vi "ContinousTest.vi"() -> ()   [LabVIEW 2020]
uses:
  <vilib>/Analysis/NI_AALBase.lvlib
  source/library/openg_md5.lvlib
  source/library/MD5 Message Digest/MD5 Message Digest (Binary String).vi
panel:
  out "Iteration":i32
  out "All OK?":bool
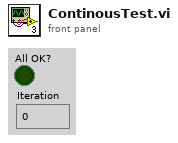
[diagram p1: front panel]
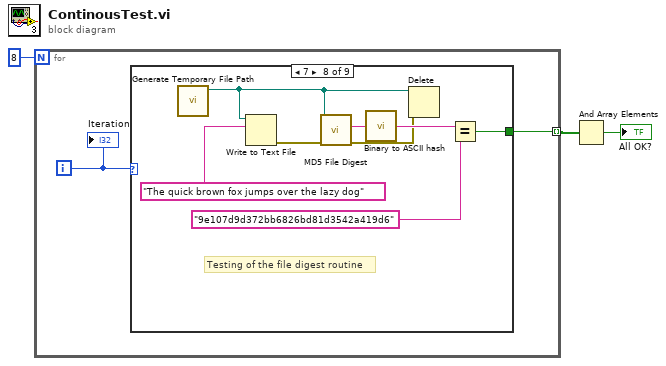
[diagram p0: block diagram]
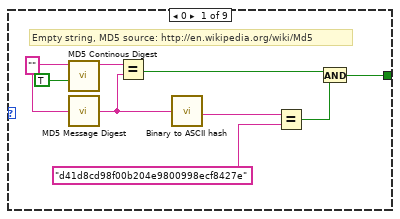
[diagram p2: hidden frame]
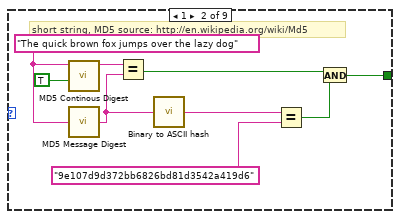
[diagram p3: hidden frame]
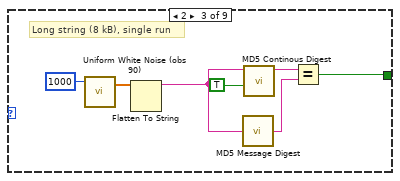
[diagram p4: hidden frame]
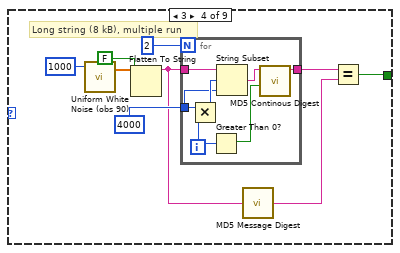
[diagram p5: hidden frame]
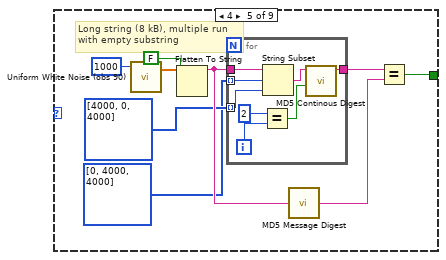
[diagram p6: hidden frame]
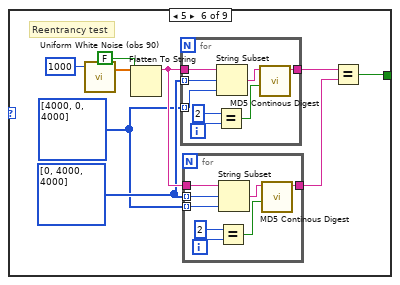
[diagram p7: hidden frame]
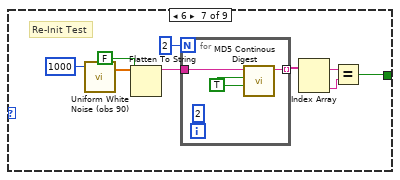
[diagram p8: hidden frame]
diagram:
  n1 = for {
    N: 8 -> [_]
    tunnel: [w4] -> w2 mode=indexing
    i -> [w5]
    n2 = case shown="7" w5 {
      tunnel: [w8 w18 w24 w35 w51 w69 w95 w101 _] -> w4
      frame 0 {
        w7 = "" ("f")
        # "Empty string, MD5 source: http://en.wikipedia.org/wiki/Md5"
        n3 = call "MD5 Continous Digest.vi"("Finish?"=TRUE, "String"=w7) -> ("MD5 Message Digest"=w13:string)  [unwired: 8 in, 1 out]
        n4 = call-poly "MD5 Message Digest.vi"("Message"=w7) -> ("MD5 Message Digest"=w6:string)
        n5 = Equal?(x=w13, y=w6) -> (x = y?=w10:bool)
        n6 = call "Binary to ASCII hash.vi"("Binary hash string"=w6) -> ("ASCII hash string"=w12:string)
        n7 = Equal?(x=w12, y="d41d8cd98f00b204e9800998ecf8427e") -> (x = y?=w9:bool)
        n8 = And(x=w10, y=w9) -> (x .and. y?=w8:bool)
      }
      frame 1 {
        w16 = "The quick brown fox jumps over the lazy dog" ("f")
        # "short string, MD5 source: http://en.wikipedia.org/wiki/Md5"
        n9 = call "MD5 Continous Digest.vi"("Finish?"=TRUE, "String"=w16) -> ("MD5 Message Digest"=w22:string)  [unwired: 8 in, 1 out]
        n10 = call-poly "MD5 Message Digest.vi"("Message"=w16) -> ("MD5 Message Digest"=w15:string)
        n11 = Equal?(x=w22, y=w15) -> (x = y?=w20:bool)
        n12 = call "Binary to ASCII hash.vi"("Binary hash string"=w15) -> ("ASCII hash string"=w17:string)
        n13 = Equal?(x=w17, y="9e107d9d372bb6826bd81d3542a419d6") -> (x = y?=w19:bool)
        n14 = And(x=w20, y=w19) -> (x .and. y?=w18:bool)
      }
      frame 2 {
        # "Long string (8 kB), single run"
        n15 = call <vilib>:"Uniform White Noise (obs 90).vi"("samples"=1000) -> ("uniform white noise"=w26:dbl[])  [unwired: 2 in, 1 out]
        n16 = Flatten To String(anything=w26) -> (data string=w25:string)  [unwired: 3 in, 2 out]
        n17 = call-poly "MD5 Message Digest.vi"("Message"=w25) -> ("MD5 Message Digest"=w28:string)
        n18 = call "MD5 Continous Digest.vi"("Finish?"=TRUE, "String"=w25) -> ("MD5 Message Digest"=w29:string)  [unwired: 8 in, 1 out]
        n19 = Equal?(x=w29, y=w28) -> (x = y?=w24:bool)
      }
      frame 3 {
        # "Long string (8 kB), multiple run"
        n20 = call <vilib>:"Uniform White Noise (obs 90).vi"("samples"=1000) -> ("uniform white noise"=w36:dbl[])  [unwired: 2 in, 1 out]
        n21 = Flatten To String(anything=w36, prepend array or string size? (T)=FALSE) -> (data string=w31:string)  [unwired: 2 in, 2 out]
        n22 = for {
          N: 2 -> [_]
          tunnel: [w46] -> w39
          tunnel: w31 -> [w45]
          tunnel: 4000 -> [w42]
          i -> [w44]
          n23 = Multiply(x=w42, y=w44) -> (x*y=w43:i32)
          n24 = Greater Than 0?(x=w44) -> (x > 0?=w40:bool)
          n25 = String Subset(string=w45, offset (0)=w43, length (rest)=w42) -> (substring=w41:string)
          n26 = call "MD5 Continous Digest.vi"("Finish?"=w40, "String"=w41) -> ("MD5 Message Digest"=w46:string)  [unwired: 8 in, 1 out]
        }
        n27 = call-poly "MD5 Message Digest.vi"("Message"=w31) -> ("MD5 Message Digest"=w38:string)
        n28 = Equal?(x=w39, y=w38) -> (x = y?=w35:bool)
      }
      frame 4 {
        # "Long string (8 kB), multiple run\nwith empty substring"
        n29 = call <vilib>:"Uniform White Noise (obs 90).vi"("samples"=1000) -> ("uniform white noise"=w52:dbl[])  [unwired: 2 in, 1 out]
        n30 = Flatten To String(anything=w52, prepend array or string size? (T)=FALSE) -> (data string=w49:string)  [unwired: 2 in, 2 out]
        n31 = for {
          tunnel: [w63] -> w55
          tunnel: w49 -> [w62]
          tunnel: i32[] [4000, 0, 4000] -> [w60] mode=indexing
          tunnel: i32[] [0, 4000, 4000] -> [w59] mode=indexing
          i -> [w58]
          n32 = Equal?(x=2, y=w58) -> (x = y?=w57:bool)
          n33 = String Subset(string=w62, offset (0)=w59, length (rest)=w60) -> (substring=w61:string)
          n34 = call "MD5 Continous Digest.vi"("Finish?"=w57, "String"=w61) -> ("MD5 Message Digest"=w63:string)  [unwired: 8 in, 1 out]
        }
        n35 = call-poly "MD5 Message Digest.vi"("Message"=w49) -> ("MD5 Message Digest"=w54:string)
        n36 = Equal?(x=w55, y=w54) -> (x = y?=w51:bool)
      }
      frame 5 {
        w65 = i32[] [0, 4000, 4000]
        w64 = i32[] [4000, 0, 4000]
        # "Reentrancy test"
        n37 = call <vilib>:"Uniform White Noise (obs 90).vi"("samples"=1000) -> ("uniform white noise"=w70:dbl[])  [unwired: 2 in, 1 out]
        n38 = Flatten To String(anything=w70, prepend array or string size? (T)=FALSE) -> (data string=w66:string)  [unwired: 2 in, 2 out]
        n39 = for {
          tunnel: [w88] -> w72
          tunnel: w66 -> [w87]
          tunnel: w64 -> [w85] mode=indexing
          tunnel: w65 -> [w84] mode=indexing
          i -> [w83]
          n40 = Equal?(x=2, y=w83) -> (x = y?=w82:bool)
          n41 = String Subset(string=w87, offset (0)=w84, length (rest)=w85) -> (substring=w86:string)
          n42 = call "MD5 Continous Digest.vi"("Finish?"=w82, "String"=w86) -> ("MD5 Message Digest"=w88:string)  [unwired: 8 in, 1 out]
        }
        n43 = for {
          tunnel: [w80] -> w67
          tunnel: w66 -> [w79]
          tunnel: w64 -> [w77] mode=indexing
          tunnel: w65 -> [w76] mode=indexing
          i -> [w75]
          n44 = Equal?(x=2, y=w75) -> (x = y?=w74:bool)
          n45 = String Subset(string=w79, offset (0)=w76, length (rest)=w77) -> (substring=w78:string)
          n46 = call "MD5 Continous Digest.vi"("Finish?"=w74, "String"=w78) -> ("MD5 Message Digest"=w80:string)  [unwired: 8 in, 1 out]
        }
        n47 = Equal?(x=w72, y=w67) -> (x = y?=w69:bool)
      }
      frame 6 {
        # "Re-Init Test"
        n48 = call <vilib>:"Uniform White Noise (obs 90).vi"("samples"=1000) -> ("uniform white noise"=w96:dbl[])  [unwired: 2 in, 1 out]
        n49 = Flatten To String(anything=w96, prepend array or string size? (T)=FALSE) -> (data string=w93:string)  [unwired: 2 in, 2 out]
        n50 = for {
          N: 2 -> [_]
          tunnel: [w100] -> w92 mode=indexing
          tunnel: w93 -> [w98]
          w99 = TRUE ("Finish?")
          (unwired) 2 ("x")
          n51 = call "MD5 Continous Digest.vi"("Finish?"=w99, "ReInit?"=w99, "String"=w98) -> ("MD5 Message Digest"=w100:string)  [unwired: 7 in, 1 out]
        }
        n52 = Index Array(array=w92) -> (element #1=w91:string, element #2=w90:string)  [unwired: 2 in]
        n53 = Equal?(x=w91, y=w90) -> (x = y?=w95:bool)
      }
      frame 7 {
        # "Testing of the file digest routine"
        n54 = call <vilib>:"Generate Temporary File Path.vi"() -> ("Unique Temporary File Path"=w102:path)  [unwired: 10 in, 1 out]
        n55 = Write to Text File(file (use dialog)=w102, text="The quick brown fox jumps over the lazy dog" ("f")) -> (error out=w107:errorcluster)  [unwired: 2 in, 2 out]
        n56 = call "MD5 File Digest.vi"("error in (no error)"=w107, "File"=w102) -> ("error out"=w103:errorcluster, "MD5 hash"=w106:string)  [unwired: 8 in]
        n57 = call "Binary to ASCII hash.vi"("Binary hash string"=w106) -> ("ASCII hash string"=w105:string)
        n58 = Delete(path (use dialog)=w102, error in=w103) -> ()  [unwired: 3 in, 3 out]
        n59 = Equal?(x=w105, y="9e107d9d372bb6826bd81d3542a419d6") -> (x = y?=w101:bool)
      }
      frame Default {
      }
    }
    "Iteration" <- w5
  }
  n60 = And Array Elements(Boolean array=w2) -> (logical AND=→"All OK?":bool)
